vi "Start.vi"(8 "error in (no error)":errorcluster, 11 "1553 Component in":refnum<class "1553 Component.lvclass">) -> (0 "error out":errorcluster, 3 "1553 Component out":refnum<class "1553 Component.lvclass">)   [LabVIEW 2020, in "BCI-1553 API.lvlib" / "1553 Component.lvclass"]
doc: "Starts the operation of a component after it has been configured."
uses:
  1553 Component.lvclass
  1553 Component.lvclass/1553 Component.ctl
  1553 SubComponent/1553 SubComponent.lvclass
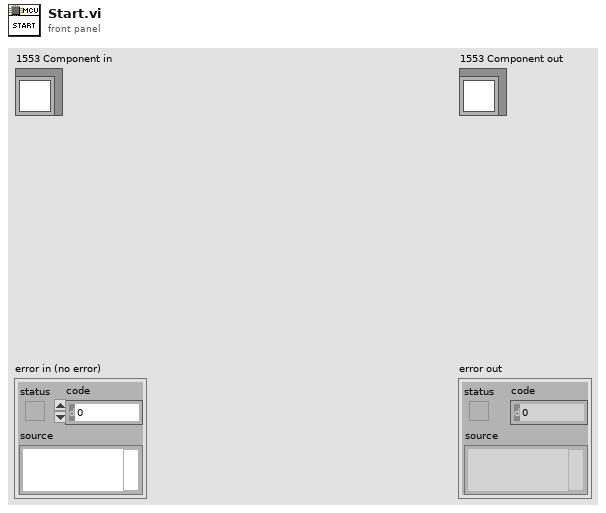
[diagram p1: front panel]
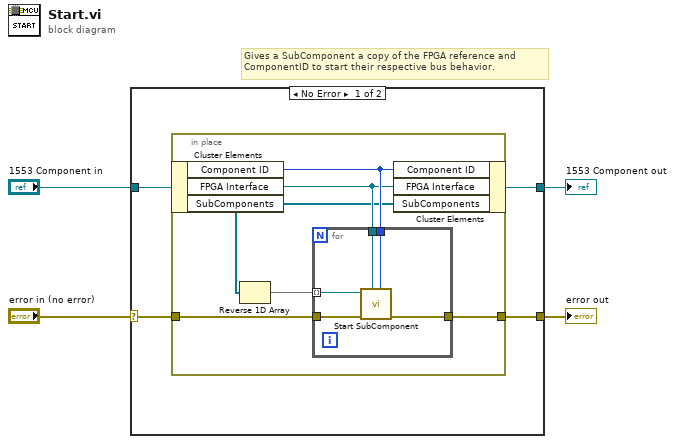
[diagram p0: block diagram]
diagram:
  # "Gives a SubComponent a copy of the FPGA reference and\nComponentID to start their respective bus behavior."
  n1 = case shown="No Error" "error in (no error)" {
    selector: "error in (no error)" -> [w8 w21]
    tunnel: [w7 w21] -> w3
    tunnel: [w5 w20] -> w1
    tunnel: "1553 Component in" -> [w6 w20]
    frame No Error {
      n2 = in-place {
        in-place-border: w8 -> [w14]
        in-place-border: [w13] -> w7
        n3 = in-place-cluster #1(w6) -> ("Component ID"=w12:u8, "FPGA Interface"=w11:refnum<class "FPGA Interface.lvclass">, "SubComponents"=w10:refnum<class "1553 SubComponent.lvclass">[])
        n4 = Reverse 1D Array(array=w10) -> (reversed array=w9:refnum<class "1553 SubComponent.lvclass">[])
        n5 = for {
          tunnel: w9 -> [w19] mode=indexing
          tunnel: w14 -> [w18]
          tunnel: [w15] -> w13
          tunnel: w11 -> [w17]
          tunnel: w12 -> [w16]
          n6 = call-dynamic "Start SubComponent.vi"("Component ID"=w16, "FPGA Interface"=w17, "error in (no error)"=w18, "1553 SubComponent in"=w19) -> ("error out"=w15:errorcluster)  [unwired: 6 in, 1 out]
        }
        n7 = in-place-cluster #1("Component ID"=w12, "FPGA Interface"=w11, "SubComponents"=w10) -> (w5:refnum<class "1553 Component.lvclass">)
      }
    }
    frame Error {
    }
  }
  "error out" <- w3
  "1553 Component out" <- w1
